vi "stageSetOrigin.vi"   [LabVIEW 2016]
uses:
  <vilib>/Instr/_visa.llb/VISA Configure Serial Port (Instr).vi
  variables/configDB.vi
  <vilib>/Utility/config.llb/Read Key (String).vi
  <vilib>/Utility/config.llb/Write Key (String).vi
  <vilib>/Utility/config.llb/NI_LVConfig.lvlib
types:
  T1 = typedef "NI_LVConfig.lvlib/Config Data RefNum.ctl" = refnum<k1>
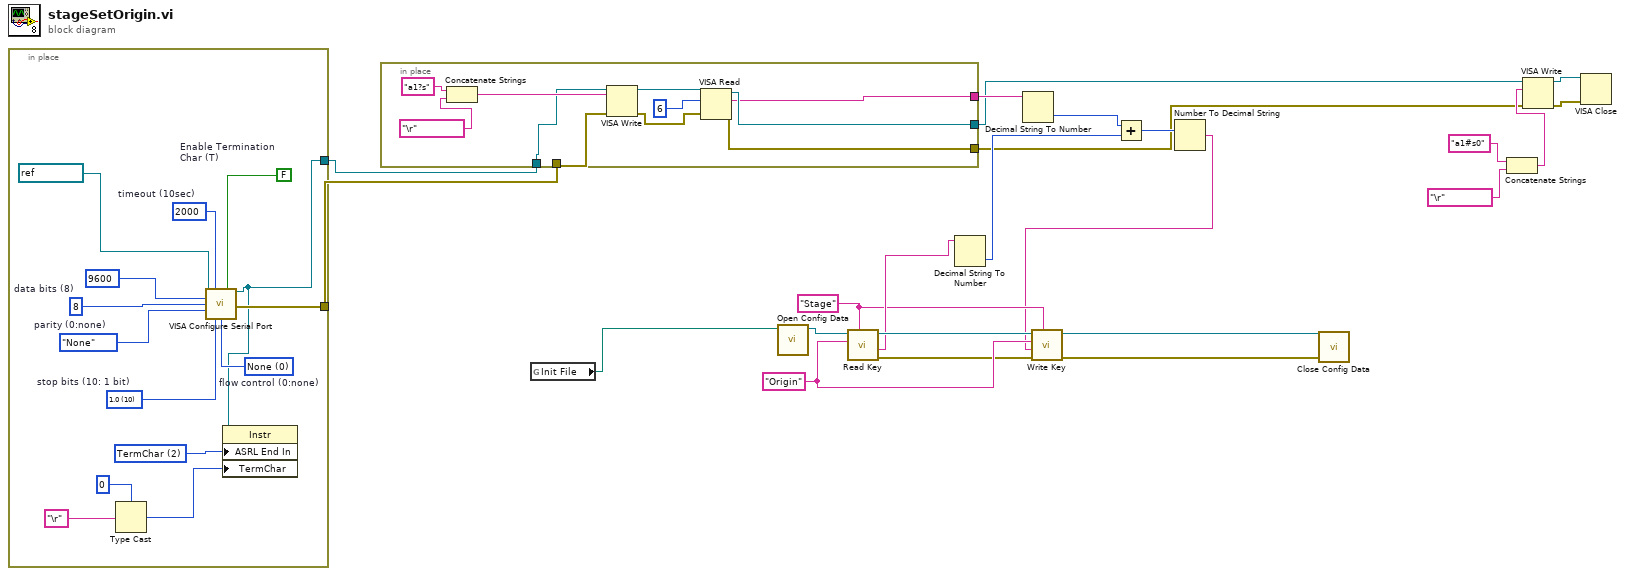
[diagram p0: block diagram]
diagram:
  w13 = "Origin" ("key")
  w14 = "Stage" ("section")
  n1 = in-place {
    in-place-border: [w24] -> w23
    in-place-border: [w29] -> w22
    w25 = u16 2 items=["None", "Last Bit", "TermChar"] ("Serial Settings:End Mode for Reads")
    w31 = u16 0 items=["None", "XON/XOFF", "RTS/CTS", "XON/XOFF & RTS/CTS", "DTR/DSR", "XON/XOFF & DTR/DSR"]  # flow control (0:none)
    w32 = u16 10 items=["1.0"=10, "1.5"=15, "2.0"=20]  # stop bits (10: 1 bit)
    w33 = FALSE  # Enable Termination Char (T)
    w34 = u32 2000  # timeout (10sec)
    w35 = enum16{"None", "Odd", "Even", "Mark", "Space"}."None"  # parity (0:none)
    w36 = u16 8  # data bits (8)
    n2 = Type Cast(type=u8 0, x="\r") -> (*(type *) &x=w27:u8)
    n3 = call-poly "VISA Configure Serial Port"("VISA resource name"=refnum<visa-resource-name> "COM4", "timeout (10sec)"=w34, "Enable Termination\nChar (T)"=w33, "baud rate (9600)"=u32 9600, "data bits (8)"=w36, "parity (0:none)"=w35, "stop bits (10: 1 bit)"=w32, "flow control (0:none)"=w31) -> ("VISA resource name out"=w24:refnum<visa-resource-name>, "error out"=w29:errorcluster)  [unwired: 6 in]
    n4 = property class="Instr"(reference=w24, "ASRL End In"=w25, "TermChar"=w27) -> ()  [unwired: 1 in, 2 out]
  }
  n5 = in-place {
    in-place-border: w23 -> [w43]
    in-place-border: w22 -> [w42]
    in-place-border: [w41] -> w2
    in-place-border: [w40] -> w3
    in-place-border: [w38] -> w19
    n6 = Concatenate Strings("a1?s" ("write buffer"), "\r" ("write buffer")) -> (w46:string)
    n7 = VISA Write(VISA resource name=w43, write buffer=w46, error in (no error)=w42) -> (VISA resource name out=w47:refnum<visa-resource-name>, error out=w39:errorcluster)  [unwired: 1 out]
    n8 = VISA Read(VISA resource name=w47, byte count=u32 6, error in (no error)=w39) -> (VISA resource name out=w40:refnum<visa-resource-name>, read buffer=w38:string, error out=w41:errorcluster)  [unwired: 1 out]
  }
  n9 = global read "configDB.vi" "Init File"() -> (w1:path)
  n10 = call <vilib>:"Open Config Data.vi"("configuration file path"=w1) -> ("refnum"=w21:T1)  [unwired: 8 in, 2 out]
  n11 = call-poly <vilib>:"Read Key.vi"("section"=w14, "key"=w13, "refnum"=w21) -> ("error out"=w12:errorcluster, "value"=w18:string, "refnum out"=w20:T1)  [unwired: 5 in, 1 out]
  n12 = Decimal String To Number(string=w18) -> (number=w16:i32)  [unwired: 2 in, 1 out]
  n13 = Decimal String To Number(string=w19) -> (number=w17:i32)  [unwired: 2 in, 1 out]
  n14 = Add(x=w17, y=w16) -> (x+y=w10:i32)
  n15 = Number To Decimal String(number=w10) -> (decimal integer string=w9:string)  [unwired: 1 in]
  n16 = call-poly <vilib>:"Write Key.vi"("section"=w14, "error in (no error)"=w12, "value"=w9, "key"=w13, "refnum"=w20) -> ("error out"=w11:errorcluster, "refnum out"=w15:T1)  [unwired: 4 in, 1 out]
  n17 = call <vilib>:"Close Config Data.vi"("error in (no error)"=w11, "refnum"=w15) -> ()  [unwired: 8 in, 2 out]
  n18 = Concatenate Strings("a1#s0", "\r" ("write buffer")) -> (w4:string)
  n19 = VISA Write(VISA resource name=w3, write buffer=w4, error in (no error)=w2) -> (VISA resource name out=w8:refnum<visa-resource-name>, error out=w7:errorcluster)  [unwired: 1 out]
  n20 = VISA Close(VISA resource name=w8, error in (no error)=w7) -> ()  [unwired: 1 out]
